vi "Go to field (PID) (No Objects).vi"(8 "error in (no error)":errorcluster, 10 "Desired Field":dbl[unit], 11 "Varian Magnet In":T2={"Fluke VISA resource name"="GPIB0::2::INSTR", "DAQ Physical Channel"="Dev1/ao0", "DAQ Task - Set"="", "DAQ Task - Read"="", "Control Voltage"=enum."40V", "extrapolated"={"x locations"=[], "coefficients"=[]}, "last 5 field numbers"=[], "Fluke Multimeter"={"function (0:volts DC)"=0, "range (0:auto)"=0, "rate (0:slow)"=0, "trigger mode (0:internal)"=0, "Autorange"=FALSE}} {"extrapolated"."x locations" format="%.4g"; "extrapolated"."coefficients" format="%.4g"; "Fluke Multimeter"."function (0:volts DC)" items=["volts DC", "volts AC", "2-wire k.ohms", "4-wire k.ohms", "mA DC", "mA AC"]; "Fluke Multimeter"."range (0:auto)" items=["autorange", "200mV, 200 ohms", "2V, 2 kohms", "20V, 20 kohms", "200V, 200 kohms", "1000Vdc, 700 Vac, 2 Mohms", "20 Mohms"]; "Fluke Multimeter"."rate (0:slow)" items=["slow", "medium", "fast"]; "Fluke Multimeter"."trigger mode (0:internal)" items=["internal - continuous trigger", "external - rear panel trigger with delay", "external - bus trigger with delay", "external - rear panel trigger", "external - bus trigger"]}) -> (0 "error out":errorcluster, 1 "Control Voltage":dbl, 2 "Current Field":dbl[unit], 3 "Varian Magnet Out":T2={"Fluke VISA resource name"="GPIB0::2::INSTR", "DAQ Physical Channel"="Dev1/ao0", "DAQ Task - Set"="", "DAQ Task - Read"="", "Control Voltage"=enum."40V", "extrapolated"={"x locations"=[], "coefficients"=[]}, "last 5 field numbers"=[], "Fluke Multimeter"={"function (0:volts DC)"=0, "range (0:auto)"=0, "rate (0:slow)"=0, "trigger mode (0:internal)"=0, "Autorange"=FALSE}} {"extrapolated"."x locations" format="%.4g"; "extrapolated"."coefficients" format="%.4g"; "Fluke Multimeter"."function (0:volts DC)" items=["volts DC", "volts AC", "2-wire k.ohms", "4-wire k.ohms", "mA DC", "mA AC"]; "Fluke Multimeter"."range (0:auto)" items=["autorange", "200mV, 200 ohms", "2V, 2 kohms", "20V, 20 kohms", "200V, 200 kohms", "1000Vdc, 700 Vac, 2 Mohms", "20 Mohms"]; "Fluke Multimeter"."rate (0:slow)" items=["slow", "medium", "fast"]; "Fluke Multimeter"."trigger mode (0:internal)" items=["internal - continuous trigger", "external - rear panel trigger with delay", "external - bus trigger with delay", "external - rear panel trigger", "external - bus trigger"]})   [LabVIEW 2009]
doc: "Uses a PID controller to maintain field at desired value. Uses last 5 field points from member data to record previous points."
uses:
  <vilib>/gmath/interp.llb/in_piecewise interp poly control.ctl
  Varian/Varian.lvlib
  <vilib>/gmath/NI_Gmath.lvlib
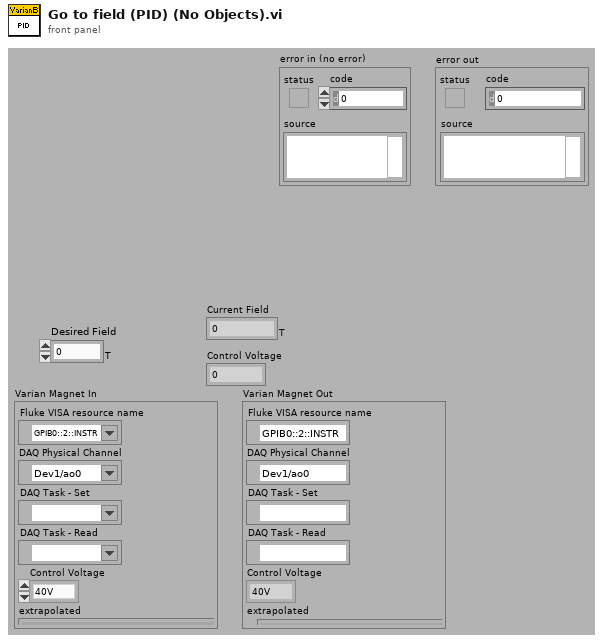
[diagram p1: front panel]
types:
  T1 = typedef "NI_Gmath.lvlib/in_piecewise interp poly control.ctl" = cluster{"x locations":dbl[], "coefficients":dbl[][]}
  T2 = cluster{"Fluke VISA resource name":refnum<visa-resource-name>, "DAQ Physical Channel":tag, "DAQ Task - Set":refnum<k21>, "DAQ Task - Read":refnum<k21>, "Control Voltage":enum16{"Please Select a Value", "30V", "40V"}, "extrapolated":T1, "last 5 field numbers":dbl[], "Fluke Multimeter":cluster{"function (0:volts DC)":u16, "range (0:auto)":u16, "rate (0:slow)":u16, "trigger mode (0:internal)":u16, "Autorange":bool}}
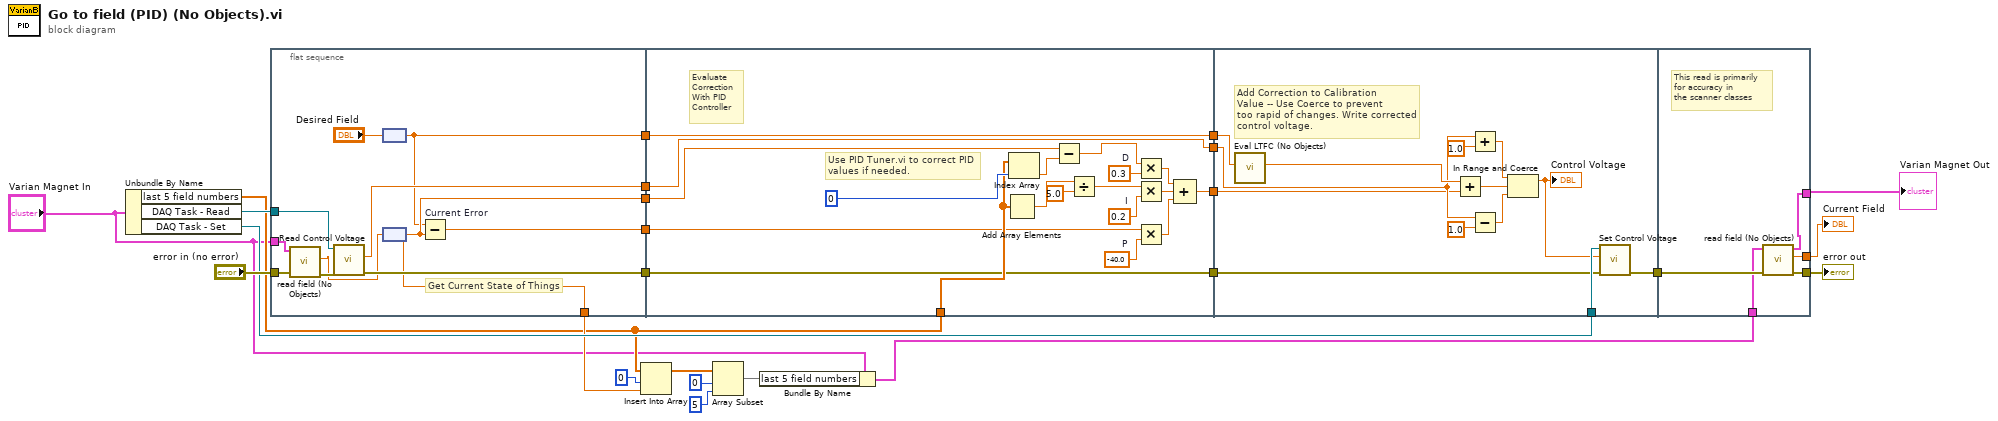
[diagram p0: block diagram]
diagram:
  n1 = Unbundle By Name("Varian Magnet In") -> ("last 5 field numbers"=w11:dbl[], "DAQ Task - Read"=w20:refnum<k21>, "DAQ Task - Set"=w16:refnum<k21>)
  n2 = flat-sequence {
    tunnel: "Varian Magnet In" -> [w26]
    tunnel: "error in (no error)" -> [w29]
    tunnel: [w36] -> w24
    tunnel: [w32] -> w23
    tunnel: [w31] -> w21
    tunnel: w20 -> [w35]
    tunnel: [w34] -> w18
    tunnel: [w33] -> w14
    tunnel: [w32] -> w13
    tunnel: w11 -> [w52]
    tunnel: w24 -> [w49]
    tunnel: w23 -> [w50]
    tunnel: [w40] -> w22
    tunnel: w21 -> [w40]
    tunnel: [w39] -> w19
    tunnel: w18 -> [w39]
    tunnel: [w38] -> w17
    tunnel: [w37] -> w15
    tunnel: w14 -> [w37]
    tunnel: w22 -> [w68]
    tunnel: w19 -> [w65]
    tunnel: w17 -> [w60]
    tunnel: w16 -> [w59]
    tunnel: w15 -> [w58]
    tunnel: [w57] -> w6
    tunnel: w6 -> [w72]
    tunnel: [w73] -> w5
    tunnel: w4 -> [w71]
    tunnel: [w70] -> w1
    tunnel: [w69] -> w3
    frame #0 {
      # "Get Current State of Things"
      n3 = call "read field (No Objects).vi"("error in (no error)"=w29, "Varian Magnet In"=w26) -> ("error out"=w28:errorcluster, "Field"=w27:dbl[unit])  [unwired: 7 in, 1 out]
      n4 = call "Read Control Voltage.vi"("error in"=w28, "task in"=w35) -> ("error out"=w33:errorcluster, "Current Control Voltage"=w34:dbl)  [unwired: 7 in, 1 out]
      n5 = node("Desired Field") -> (w31:dbl)
      n6 = node(w27) -> (w32:dbl)
      n7 = Subtract "Current Error"(x=w31, y=w32) -> (x-y=w36:dbl)
    }
    frame #1 {
      w48 = -40.0  # P
      w44 = 0.3  # D
      w46 = 0.2  # I
      # "Use PID Tuner.vi to correct PID\nvalues if needed."
      # "Evaluate\nCorrection\nWith PID\nController"
      n8 = Add Array Elements(numeric array=w52) -> (sum=w55:dbl)
      n9 = Index Array(array=w52, index=0) -> (element=w54:dbl)
      n10 = Subtract(x=w50, y=w54) -> (x-y=w45:dbl)
      n11 = Divide(x=w55, y=5.0) -> (x/y=w47:dbl)
      n12 = Multiply(x=w45, y=w44) -> (x*y=w43:dbl)
      n13 = Multiply(x=w47, y=w46) -> (x*y=w42:dbl)
      n14 = Multiply(x=w49, y=w48) -> (x*y=w41:dbl)
      n15 = Compound Arithmetic op=ADD(w43, w42, w41) -> (w38:dbl)
    }
    frame #2 {
      # "Add Correction to Calibration\nValue -- Use Coerce to prevent\ntoo rapid of changes. Write corrected\ncontrol voltage."
      n16 = call "Eval LTFC (No Objects).vi"("Desired Field (T)"=w68) -> ("Desired Control Voltage"=w67:dbl)  [unwired: 9 in, 1 out]
      n17 = Add(x=w67, y=w60) -> (x+y=w66:dbl)
      n18 = Add(x=w65, y=1.0) -> (x+y=w61:dbl)
      n19 = Subtract(x=w65, y=1.0) -> (x-y=w62:dbl)
      n20 = In Range and Coerce(upper limit=w61, x=w66, lower limit=w62) -> (coerced(x)=w56:dbl)  [unwired: 1 out]
      "Control Voltage" <- w56
      n21 = call "Set Control Voltage.vi"("error in"=w58, "Control Voltage"=w56, "task in"=w59) -> ("error out"=w57:errorcluster)  [unwired: 8 out]
    }
    frame #3 {
      # "This read is primarily\nfor accuracy in\nthe scanner classes"
      n22 = call "read field (No Objects).vi"("error in (no error)"=w72, "Varian Magnet In"=w71) -> ("error out"=w73:errorcluster, "Field"=w69:dbl[unit], "Varian Magnet Out"=w70:T2)  [unwired: 7 in]
    }
  }
  n23 = Insert Into Array(array=w11, index=0, new element=w13) -> (w10:dbl[])
  n24 = Array Subset(array=w10, index=0, length=5) -> (w7:dbl[])
  n25 = Bundle By Name(cluster="Varian Magnet In", "last 5 field numbers"=w7) -> (w4:T2)
  "error out" <- w5
  "Current Field" <- w3
  "Varian Magnet Out" <- w1
